vi "Backlight Value.vi"(10 "Backlight":bool) -> (2 "BacklightVal":u8)   [LabVIEW 2023, in "CTI-Visa-DeviceLib.lvlib" / "LCD-I2C.lvclass"]
uses:
  LCD-I2C.lvclass
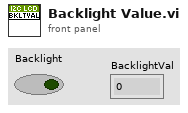
[diagram p1: front panel]
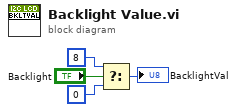
[diagram p0: block diagram]
diagram:
  n1 = Select(t=u8 8 ("BacklightVal"), s="Backlight", f=u8 0 ("BacklightVal")) -> (s? t:f=→"BacklightVal":u8)
